vi "UseEnableChannel Value Change.vi"(7 "Enable Tag ref":refnum<vi>, 10 "Use Enable Channel":bool, 11 "References":T1) -> (0 "error out":errorcluster, 2 "Enable Tag":string)   [LabVIEW 2015, in "TDMS datalogger editor node.lvclass"]
uses:
  TDMS datalogger editor node.lvclass
  <vilib>/NI/DCAF/Tag Editor Core/Table API/Table Manager/object ref.ctl
  <vilib>/NI/DCAF/Tag Editor Core/Configuration Editor/Classes/Engine Parent/Engine Parent Editor Node.lvclass
  <vilib>/NI/DCAF/Tag Editor Core/Configuration Editor/Classes/Module editor node/module editor node.lvclass
  TDMS datalogger editor node.lvclass/TDMS datalogger editor node.ctl
  <vilib>/NI/Configuration Framework/serializable configuration/NISE_CEF_serializable configuration.lvclass/NISE_CEF_serializable configuration.ctl
  module/configuration/TDMS datalogger configuration.lvclass/TDMS datalogger configuration.ctl
  <vilib>/Utility/LVClass/Get LV Class Name.vi
  <vilib>/NI/Configuration Framework/error generator/NISE_error generator.vi
  <vilib>/NI/Module Execution Interface/Engine Configuration/engine configuration.lvclass
  module/configuration/TDMS datalogger configuration.lvclass
  <vilib>/NI/Configuration Framework/serializable configuration/NISE_CEF_serializable configuration.lvclass
  <vilib>/NI/DCAF/Tag Editor Core/Table API/Table Manager/Table Manager.lvclass
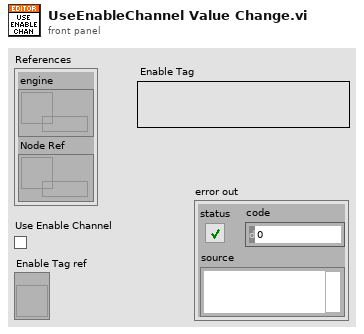
[diagram p1: front panel]
types:
  T1 = typedef "Table Manager.lvlib/Table Manager.lvclass/object ref.ctl" = cluster{"engine":refnum<data-value>, "Node Ref":refnum<data-value>}
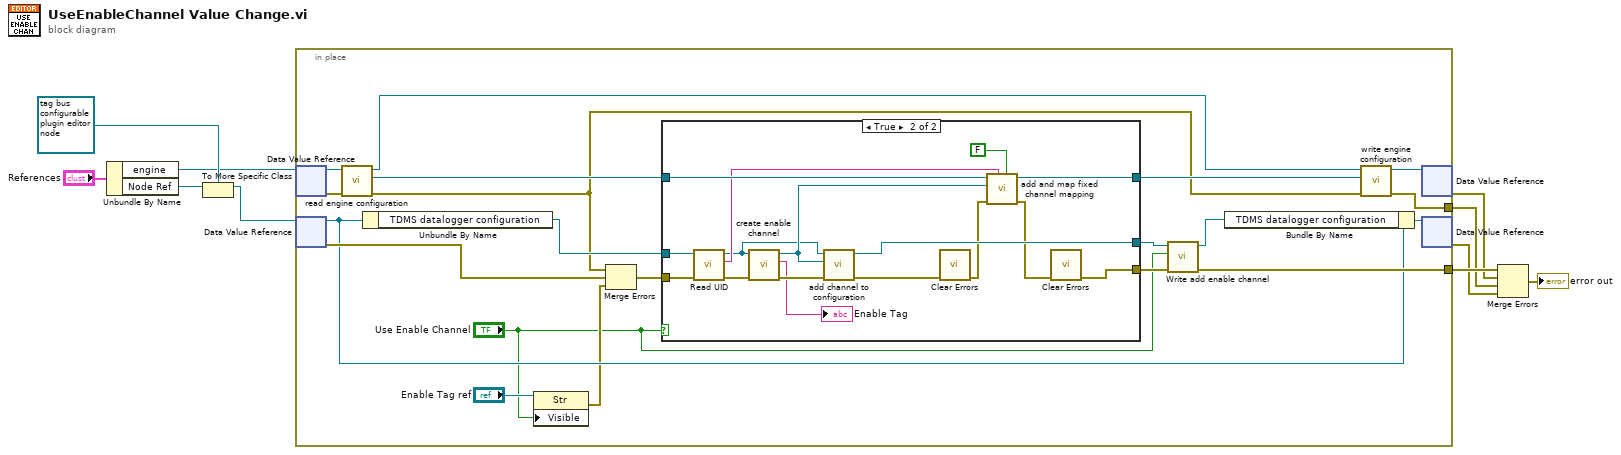
[diagram p0: block diagram]
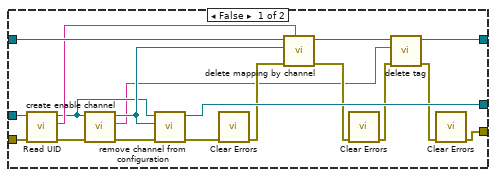
[diagram p2: hidden frame]
diagram:
  n1 = Unbundle By Name("References") -> ("engine"=w2:refnum<data-value>, "Node Ref"=w5:refnum<data-value>)
  n2 = To More Specific Class(target class=refnum<data-value> refnum ("data value reference"), reference=w5) -> (specific class reference=w3:refnum<data-value>)  [unwired: 1 in, 1 out]
  n3 = in-place {
    in-place-border: [w28] -> w10
    in-place-border: [w23] -> w7
    n4 = in-place-dvr #1(w2) -> (w27:refnum<class "Engine Parent Editor Node.lvclass">, w25:errorcluster)
    n5 = in-place-dvr #2(w3) -> (w21:refnum<class "TDMS datalogger editor node.lvclass">, w24:errorcluster)
    n6 = call <vilib>:"read engine configuration.vi"("error in"=w25, "Engine Parent Editor Node in"=w27) -> ("error out"=w15:errorcluster, "engine configuration"=w26:refnum<class "engine configuration.lvclass">, "Engine Parent Editor Node out"=w17:refnum<class "Engine Parent Editor Node.lvclass">)  [unwired: 7 in]
    n7 = Unbundle By Name(w21) -> ("TDMS datalogger configuration"=w22:refnum<class "TDMS datalogger configuration.lvclass">)
    n8 = property on="Property Node" class="Str"(reference="Enable Tag ref", "Visible"="Use Enable Channel") -> (error out=w12:errorcluster)  [unwired: 1 in, 1 out]
    n9 = Merge Errors(w15, w24, w12) -> (w14:errorcluster)
    n10 = case shown="True" "Use Enable Channel" {
      tunnel: [w43 w64] -> w16
      tunnel: w26 -> [w46 w60]
      tunnel: [w48 w63] -> w30
      tunnel: w22 -> [w34 w53]
      tunnel: [w39 w58] -> w29
      tunnel: w14 -> [w36 w55]
      frame False {
        n11 = call <vilib>:"Read UID.vi"("error in"=w36, "configuration in"=w34) -> ("error out"=w35:errorcluster, "instance id"=w33:string, "configuration out"=w32:refnum<class "TDMS datalogger configuration.lvclass">)  [unwired: 7 in]
        n12 = call "create enable channel.vi"("error in"=w35, "TDMS datalogger configuration"=w32) -> ("error out"=w47:errorcluster, "enable channel name"=w31:string, "enable channel"=w45:refnum<class "TBM channel.lvclass">)  [unwired: 7 in]
        n13 = call "remove channel from configuration.vi"("error in"=w47, "TBM channel in"=w45, "TDMS datalogger configuration in"=w32) -> ("error out"=w38:errorcluster, "TDMS datalogger configuration out"=w48:refnum<class "TDMS datalogger configuration.lvclass">)  [unwired: 7 in]
        n14 = call <vilib>:"Clear Errors.vi"("error in (no error)"=w38) -> ("error out"=w37:errorcluster)  [unwired: 5 in, 1 out]
        n15 = call <vilib>:"delete mapping by channel.vi"("owner ID"=w33, "error in"=w37, "channel"=w45, "engine configuration in"=w46) -> ("error out"=w41:errorcluster, "engine configuration out"=w44:refnum<class "engine configuration.lvclass">)  [unwired: 6 in]
        n16 = call <vilib>:"Clear Errors.vi"("error in (no error)"=w41) -> ("error out"=w42:errorcluster)  [unwired: 5 in, 1 out]
        n17 = call-dynamic "delete tag.vi"("error in"=w42, "tag name"=w31, "engine configuration in"=w44) -> ("error out"=w40:errorcluster, "engine configuration out"=w43:refnum<class "engine configuration.lvclass">)  [unwired: 7 in]
        n18 = call <vilib>:"Clear Errors.vi"("error in (no error)"=w40) -> ("error out"=w39:errorcluster)  [unwired: 5 in, 1 out]
      }
      frame True {
        n19 = call <vilib>:"Read UID.vi"("error in"=w55, "configuration in"=w53) -> ("error out"=w54:errorcluster, "instance id"=w52:string, "configuration out"=w50:refnum<class "TDMS datalogger configuration.lvclass">)  [unwired: 7 in]
        n20 = call "create enable channel.vi"("error in"=w54, "TDMS datalogger configuration"=w50) -> ("error out"=w62:errorcluster, "enable channel name"=→"Enable Tag":string, "enable channel"=w61:refnum<class "TBM channel.lvclass">)  [unwired: 7 in]
        n21 = call "add channel to configuration.vi"("error in"=w62, "TBM channel in"=w61, "TDMS datalogger configuration in"=w50) -> ("error out"=w57:errorcluster, "TDMS datalogger configuration out"=w63:refnum<class "TDMS datalogger configuration.lvclass">)  [unwired: 7 in]
        n22 = call <vilib>:"Clear Errors.vi"("error in (no error)"=w57) -> ("error out"=w56:errorcluster)  [unwired: 5 in, 1 out]
        n23 = call <vilib>:"add and map fixed channel mapping.vi"("set module as owner"=FALSE, "module instance"=w52, "error in"=w56, "fixed channel"=w61, "engine configuration in"=w60) -> ("error out"=w59:errorcluster, "engine configuration out"=w64:refnum<class "engine configuration.lvclass">)  [unwired: 5 in]
        n24 = call <vilib>:"Clear Errors.vi"("error in (no error)"=w59) -> ("error out"=w58:errorcluster)  [unwired: 5 in, 1 out]
      }
    }
    n25 = call "Write add enable channel.vi"("error in (no error)"=w29, "add enable channel"="Use Enable Channel", "TDMS datalogger configuration in"=w30) -> ("error out"=w28:errorcluster, "TDMS datalogger configuration out"=w20:refnum<class "TDMS datalogger configuration.lvclass">)  [unwired: 7 in]
    n26 = Bundle By Name(cluster=w21, "TDMS datalogger configuration"=w20) -> (w19:refnum<class "TDMS datalogger editor node.lvclass">)
    n27 = call <vilib>:"write engine configuration.vi"("error in"=w15, "engine configuration"=w16, "Engine Parent Editor Node in"=w17) -> ("error out"=w23:errorcluster, "Engine Parent Editor Node out"=w18:refnum<class "Engine Parent Editor Node.lvclass">)  [unwired: 7 in]
    n28 = in-place-dvr #1(w18) -> (w9:errorcluster)  [unwired: 1 out]
    n29 = in-place-dvr #2(w19) -> (w8:errorcluster)  [unwired: 1 out]
  }
  n30 = Merge Errors(w10, w9, w7, w8) -> (→"error out":errorcluster)
